vi "Operator Input Yes or No.vi"(8 "error in (no error)":errorcluster, 11 "Operator text":string) -> (0 "error out":errorcluster, 2 "No clicked":bool, 3 "Yes clicked":bool)   [LabVIEW 2013]
panel:
  in  "button2 clicked":bool caption="button2 clicked?"
  in  "button1 clicked":bool caption="button1 clicked?"
  out "Message":string
  # "Operator Message"
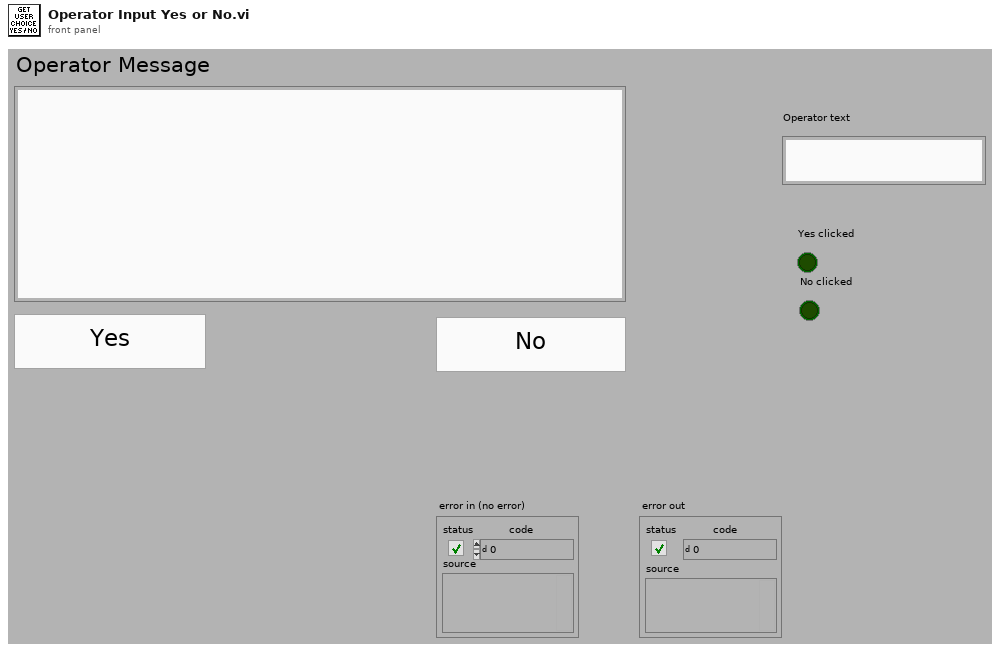
[diagram p1: front panel]
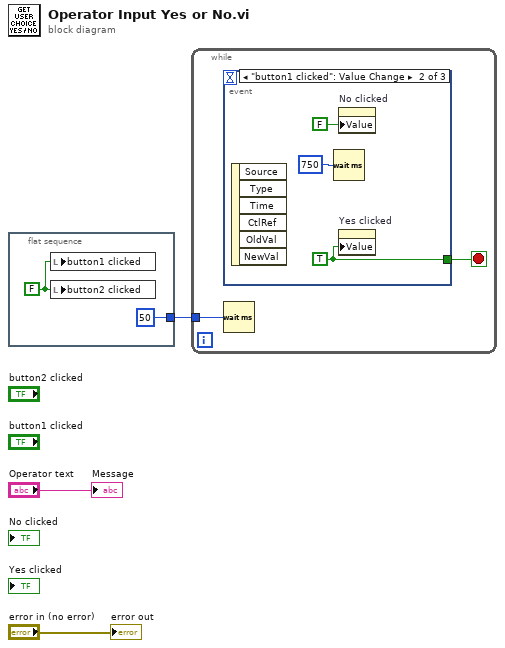
[diagram p0: block diagram]
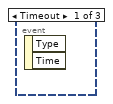
[diagram p2: hidden frame]
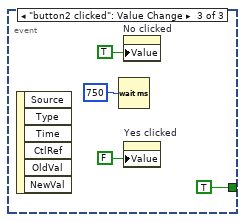
[diagram p3: hidden frame]
diagram:
  n1 = flat-sequence {
    tunnel: [u32 50 ("milliseconds to wait")] -> w3
    frame #0 {
      w4 = FALSE ("button1")
      n2 = local write "button1 clicked"(w4) -> ()
      n3 = local write "button2 clicked"(w4) -> ()
    }
  }
  n4 = while {
    tunnel: w3 -> [w7]
    stop <- w6 stop-if-true
    n5 = event shown="[1] \"button1 clicked\": Value Change" {
      selector: _ -> [_ _ _]
      dyn-events: _ -> [_ _ _]
      timeout: _ -> [_ _ _]
      tunnel: [_ w10 TRUE] -> w6
      event Timeout {
        n6 = event-data() -> ()  [unwired: 1 in, 2 out]
      }
      event "button1 clicked": Value Change {
        w10 = TRUE
        n7 = event-data() -> ()  [unwired: 1 in, 6 out]
        n8 = Wait (ms)(milliseconds to wait=u32 750) -> ()  [unwired: 1 out]
        n9 = property on="No clicked" class="Bool (strict)"("Value"=FALSE ("button2 clicked?")) -> ()  [unwired: 2 in, 2 out]
        n10 = property on="Yes clicked" class="Bool (strict)"("Value"=w10) -> ()  [unwired: 2 in, 2 out]
      }
      event "button2 clicked": Value Change {
        n11 = event-data() -> ()  [unwired: 1 in, 6 out]
        n12 = Wait (ms)(milliseconds to wait=u32 750) -> ()  [unwired: 1 out]
        n13 = property on="No clicked" class="Bool (strict)"("Value"=TRUE ("button2 clicked?")) -> ()  [unwired: 2 in, 2 out]
        n14 = property on="Yes clicked" class="Bool (strict)"("Value"=FALSE ("button1 clicked?")) -> ()  [unwired: 2 in, 2 out]
      }
    }
    n15 = Wait (ms)(milliseconds to wait=w7) -> ()  [unwired: 1 out]
  }
  "Message" <- "Operator text"
  "error out" <- "error in (no error)"
